vi "Configure Ethernet Setup.vi"(4 "Gateway IP":string="100.100.100.101", 6 "Subnet Mask (255.255.255.0)":string="255.255.255.0", 7 "Device Name (ARI 78xx)":string="ARI 78xx", 8 "error in (no error)":errorcluster, 9 "IP Address":string="100.100.100.100", 10 "IP Setup Mode":u16(ring) items=["Auto", "Manual"], 11 "VISA resource name":refnum<visa-resource-name>) -> (0 "error out":errorcluster, 3 "VISA resource name out":refnum<visa-resource-name>)   [LabVIEW 2014, in "eec EST 300.lvlib"]
doc: "Configures IP Settings for the instrument.\n1. Device Name\n2. IP Setup Mode\n3. IP Address\n4. Subnet Mask\n5. Gateway IP"
uses:
  <instrlib>/eec EST 300/eec EST 300.lvlib
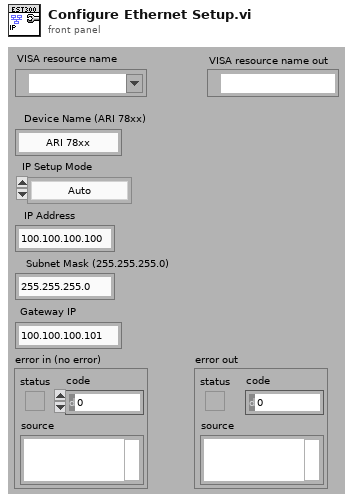
[diagram p1: front panel]
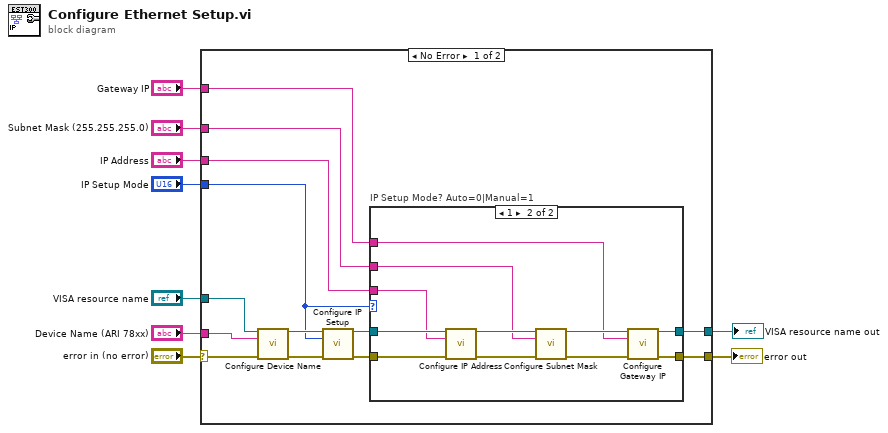
[diagram p0: block diagram]
diagram:
  n1 = case shown="No Error" "error in (no error)" {
    selector: "error in (no error)" -> [w10 w37]
    tunnel: "Device Name (ARI 78xx)" -> [w11 _]
    tunnel: "VISA resource name" -> [w22 w36]
    tunnel: "IP Setup Mode" -> [w17 _]
    tunnel: [w16 w37] -> w6
    tunnel: [w15 w36] -> w5
    tunnel: "IP Address" -> [w14 _]
    tunnel: "Subnet Mask (255.255.255.0)" -> [w13 _]
    tunnel: "Gateway IP" -> [w12 _]
    frame No Error {
      n2 = call <instrlib>:"Configure Device Name.vi"("VISA resource name"=w22, "Device Name (APT 6000)"=w11, "error in (no error)"=w10) -> ("VISA resource name out"=w21:refnum<visa-resource-name>, "error out"=w20:errorcluster)  [unwired: 11 in]
      n3 = call <instrlib>:"Configure IP Setup.vi"("VISA resource name"=w21, "IP Setup Mode (0:Auto)"=w17, "error in (no error)"=w20) -> ("VISA resource name out"=w19:refnum<visa-resource-name>, "error out"=w18:errorcluster)  [unwired: 11 in]
      n4 = case "IP Setup Mode? Auto=0|Manual=1" shown="1" w17 {
        tunnel: w19 -> [w24 w35]
        tunnel: w18 -> [w23 w34]
        tunnel: [w23 w30] -> w16
        tunnel: [w24 w29] -> w15
        tunnel: w14 -> [_ w27]
        tunnel: w13 -> [_ w26]
        tunnel: w12 -> [_ w25]
        frame 0, Default {
        }
        frame 1 {
          n5 = call <instrlib>:"Configure IP Address.vi"("VISA resource name"=w35, "IP Address"=w27, "error in (no error)"=w34) -> ("VISA resource name out"=w32:refnum<visa-resource-name>, "error out"=w33:errorcluster)  [unwired: 11 in]
          n6 = call <instrlib>:"Configure Subnet Mask.vi"("VISA resource name"=w32, "Subnet Mask (255.255.255.0)"=w26, "error in (no error)"=w33) -> ("VISA resource name out"=w28:refnum<visa-resource-name>, "error out"=w31:errorcluster)  [unwired: 11 in]
          n7 = call <instrlib>:"Configure Gateway IP.vi"("VISA resource name"=w28, "Gateway IP"=w25, "error in (no error)"=w31) -> ("VISA resource name out"=w29:refnum<visa-resource-name>, "error out"=w30:errorcluster)  [unwired: 11 in]
        }
      }
    }
    frame Error {
    }
  }
  "VISA resource name out" <- w5
  "error out" <- w6
